vi "Read_files_from_folder.vi"(8 "error in (no error)":errorcluster, 11 "Path":path) -> (0 "error out":errorcluster, 2 "Array of strings (file name, extension, size (in bytes))":string[][](array[string]), 3 "File Path":path[](array[path]))   [LabVIEW 2020]
doc: "This Vi takes <b>folder path</b> or <b>file path</b> and returns <b>array of paths</b> to the files and <b>2d array of strings</b> containg files names, extensions and sizes of the files if the file extension is .png, .jpg or .bmp. If this Vi gets as the input <b>file path</b>, which extension is neither of .png, .jpg or .bmp then dialog window will show up (informing about wrong input)."
uses:
  <vilib>/regexp/Match Regular Expression.xnode
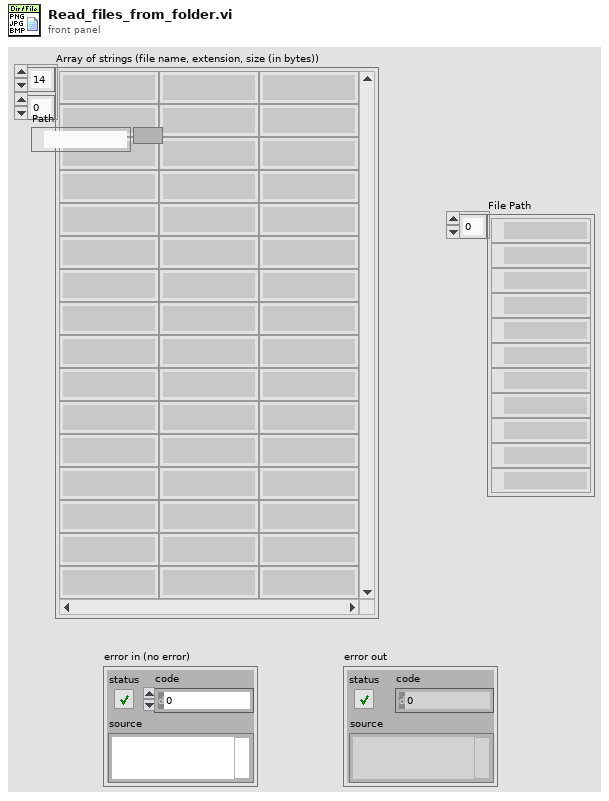
[diagram p1: front panel]
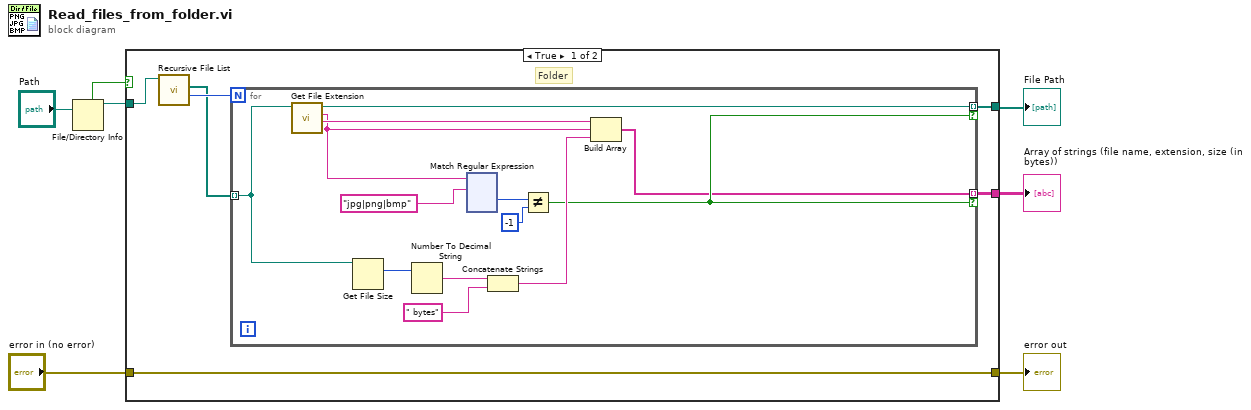
[diagram p0: block diagram]
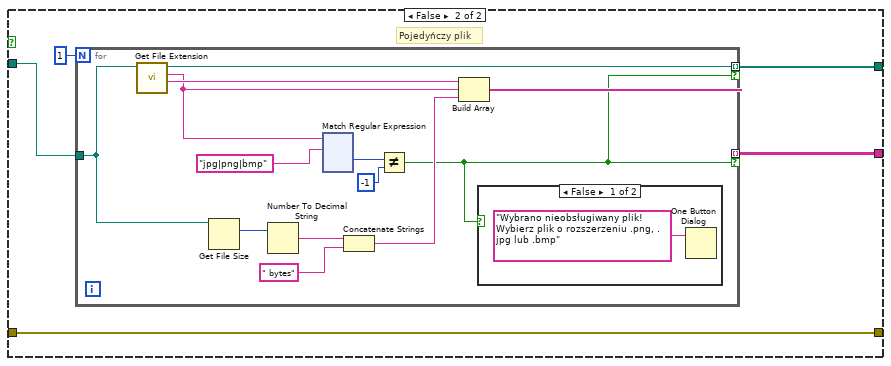
[diagram p2: hidden frame]
diagram:
  n1 = File/Directory Info(path="Path") -> (path out=w4:path, directory=w2:bool)  [unwired: 1 in, 5 out]
  n2 = case shown="True" w2 {
    tunnel: [w13 w145] -> w7
    tunnel: [w12 w144] -> w6
    tunnel: w4 -> [w9 w142]
    tunnel: "error in (no error)" -> [w8 w143]
    tunnel: [w8 w143] -> w3
    frame True {
      # "Folder"
      n3 = call <vilib>:"Recursive File List.vi"("Folder Path"=w9) -> ("Number of Files"=w11:i32, "All Files in Dir"=w10:path[])  [unwired: 6 in, 3 out]
      n4 = for {
        N: w11 -> [_]
        tunnel: w10 -> [w26] mode=indexing
        tunnel: [w14] -> w12 mode=indexing if=w16
        tunnel: [w17] -> w13 mode=indexing if=w16
        n5 = call <vilib>:"Get File Extension.vi"("file"=w26) -> ("filename without extension"=w21:string, "lowercase file extension"=w20:string, "dup file"=w17:path)  [unwired: 6 in, 2 out]
        n6 = Get File Size(file=w26) -> (size (in bytes)=w25:i64)  [unwired: 1 in, 2 out]
        n7 = Number To Decimal String(number=w25) -> (decimal integer string=w24:string)  [unwired: 1 in]
        n8 = xnode "Match Regular Expression"("input string"=w20, "regular expression"="jpg|png|bmp") -> ("offset past match"=w19:i32)  [unwired: 4 in, 4 out]
        n9 = Concatenate Strings(w24, " bytes" ("string")) -> (w22:string)
        n10 = Not Equal?(x=w19, y=-1) -> (x != y?=w16:bool)
        n11 = Build Array(w21, w20, w22) -> (w14:string[])
      }
    }
    frame False {
      # "Pojedyńczy plik"
      n12 = for {
        N: 1 -> [_]
        tunnel: w142 -> [w158]
        tunnel: [w147] -> w144 mode=indexing if=w146
        tunnel: [w149] -> w145 mode=indexing if=w146
        n13 = call <vilib>:"Get File Extension.vi"("file"=w158) -> ("filename without extension"=w153:string, "lowercase file extension"=w152:string, "dup file"=w149:path)  [unwired: 6 in, 2 out]
        n14 = Get File Size(file=w158) -> (size (in bytes)=w157:i64)  [unwired: 1 in, 2 out]
        n15 = Number To Decimal String(number=w157) -> (decimal integer string=w156:string)  [unwired: 1 in]
        n16 = xnode "Match Regular Expression"("input string"=w152, "regular expression"="jpg|png|bmp") -> ("offset past match"=w151:i32)  [unwired: 4 in, 4 out]
        n17 = Concatenate Strings(w156, " bytes" ("string")) -> (w154:string)
        n18 = Not Equal?(x=w151, y=-1) -> (x != y?=w146:bool)
        n19 = Build Array(w153, w152, w154) -> (w147:string[])
        n20 = case shown="False" w146 {
          frame False {
            n21 = One Button Dialog(message="Wybrano nieobsługiwany plik! Wybierz plik o rozszerzeniu .png, .jpg lub .bmp") -> ()  [unwired: 1 in, 1 out]
          }
          frame True {
          }
        }
      }
    }
  }
  "File Path" <- w7
  "Array of strings (file name, extension, size (in bytes))" <- w6
  "error out" <- w3
